vi "Clear.vi"(8 "error in (no error)":errorcluster, 11 "Progress in":refnum<class "Progress.lvclass">) -> (0 "error out":errorcluster)   [LabVIEW 2021, in "Progress.lvlib" / "Progress.lvclass"]
uses:
  Progress.lvclass
  5923e02f-5047-4c4b-9e21-98dd9ea94366.vi
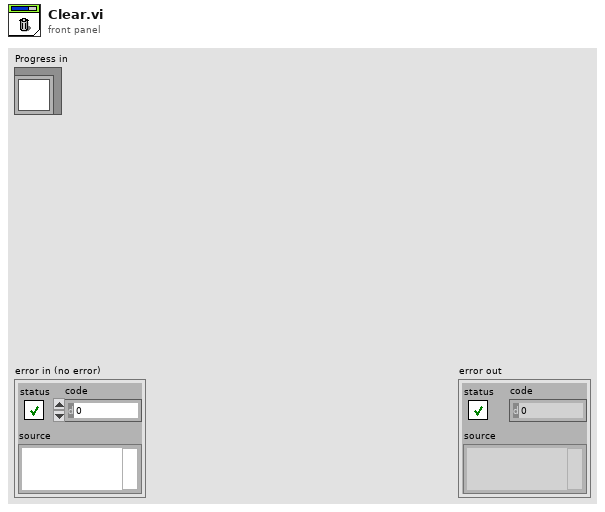
[diagram p1: front panel]
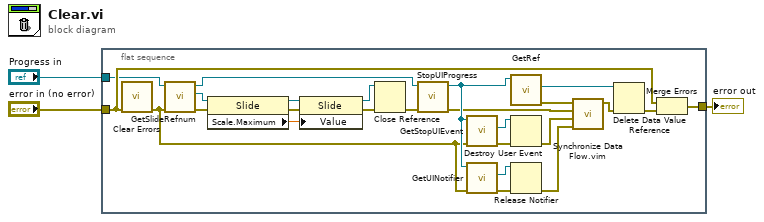
[diagram p0: block diagram]
diagram:
  n1 = flat-sequence {
    tunnel: [w28] -> w3
    tunnel: "Progress in" -> [w8]
    tunnel: "error in (no error)" -> [w27]
    frame #0 {
      n2 = call <vilib>:"Clear Errors.vi"("error in (no error)"=w27) -> ("error out"=w13:errorcluster)  [unwired: 5 in, 1 out]
      n3 = call "GetSlideRefnum.vi"("error in (no error)"=w13, "Progress in"=w8) -> ("error out"=w10:errorcluster, "SlideRefnum"=w7:refnum<vi>, "Progress out"=w9:refnum<class "Progress.lvclass">)  [unwired: 7 in]
      n4 = property class="Slide"(reference=w7, error in=w10) -> (reference out=w24:refnum<vi>, error out=w26:errorcluster, "Scale.Maximum"=w25:dbl)
      n5 = property class="Slide"(reference=w24, error in=w26, "Value"=w25) -> (reference out=w23:refnum<vi>, error out=w22:errorcluster)
      n6 = Close Reference(reference=w23, error in (no error)=w22) -> (error out=w21:errorcluster)
      n7 = call "StopUIProgress.vi"("error in (no error)"=w21, "Progress in"=w9) -> ("error out"=w12:errorcluster, "Progress out"=w20:refnum<class "Progress.lvclass">)  [unwired: 8 in]
      n8 = call "GetStopUIEvent.vi"("error in (no error)"=w13, "Progress in"=w20) -> ("error out"=w19:errorcluster, "StopUIEvent"=w18:refnum<user-event>)  [unwired: 7 in, 1 out]
      n9 = call "GetUINotifier.vi"("error in (no error)"=w13, "Progress in"=w20) -> ("error out"=w16:errorcluster, "UINotifier"=w17:refnum<notifier>)  [unwired: 7 in, 1 out]
      n10 = call "GetRef.vi"("Progress in"=w20) -> ("error out"=w11:errorcluster, "ref"=w4:refnum<data-value>)  [unwired: 8 in, 1 out]
      n11 = Destroy User Event(user event=w18, error in=w19) -> (error out=w15:errorcluster)
      n12 = Release Notifier(notifier=w17, error in (no error)=w16) -> (error out=w14:errorcluster)  [unwired: 1 in, 2 out]
      n13 = call "Synchronize Data Flow.vim"("input 4"=w14, "input 3"=w15, "input 2"=w12, "input 1"=w11) -> ("output 1"=w6:errorcluster)  [unwired: 3 out]
      n14 = Delete Data Value Reference(data value reference=w4, error in=w6) -> (error out=w5:errorcluster)  [unwired: 1 out]
      n15 = Merge Errors(w27, w5) -> (w28:errorcluster)
    }
  }
  "error out" <- w3
